vi "Trigger.vi"(2 "Enum":enum16{"Falling", "Rising", "Both"}(ring), 7 "Button":bool) -> (8 "Trigger":bool)   [LabVIEW 2016]
doc: "Rising mode - When the input changes from false to true the trigger terminal sends true for a single cycle\n\nFalling mode - When the input changes from true to false the trigger terminal sends true for a single cycle\n\nBoth mode - When the input changes the VI sends out a single pulse of true.\n\nCreated by Team 4130 for use in the 2016-2017 FRC season"
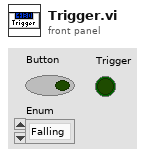
[diagram p1: front panel]
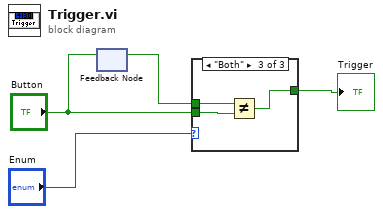
[diagram p0: block diagram]
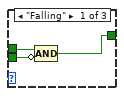
[diagram p2: hidden frame]
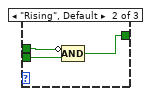
[diagram p3: hidden frame]
diagram:
  n1 = feedback #1() -> (w1:bool)  [unwired: 1 in]
  n2 = feedback-in #1("Button") -> ()
  n3 = case shown="\"Both\"" "Enum" {
    tunnel: [w5 w8 w11] -> w3
    tunnel: "Button" -> [w6 w10 w12]
    tunnel: w1 -> [w7 w9 w13]
    frame "Falling" {
      n4 = Compound Arithmetic op=AND(w7, invert w6) -> (w5:bool)
    }
    frame "Rising", Default {
      n5 = Compound Arithmetic op=AND(invert w9, w10) -> (w8:bool)
    }
    frame "Both" {
      n6 = Not Equal?(x=w13, y=w12) -> (x != y?=w11:bool)
    }
  }
  "Trigger" <- w3
